vi "cm2nm_center_fids_by_mass.vi"(1 "Array 2":i32[](array[numeric]), 2 "CollectionOfPoints":T1[](array[typedef])) -> (0 "Centered and Scaled":cluster{"X":dbl, "Y":dbl, "Z":dbl}[](array[cluster]))   [LabVIEW 2011]
doc: "Center of mass of the fiducials on the origin and scale by the distance from the origin to the furthest fiducial. Could have alternatively fit to a circle but possibly the fiducials will be not be on a circumference of a circle."
uses:
  cm2nm_coordinate_information_v2.ctl
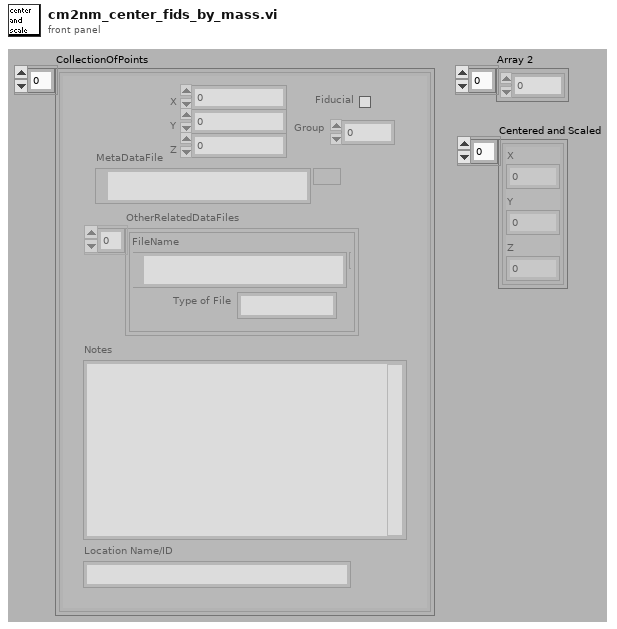
[diagram p1: front panel]
types:
  T1 = typedef "cm2nm_coordinate_information_v2.ctl" = cluster{"MetaDataFile":path, "X":dbl, "Y":dbl, "Z":dbl, "Group":i32, "Rotation":dbl[unit], "Fiducial":bool, "Magnification":dbl, "Working_Distance":dbl, "Notes":string, "Location Name/ID":string, "OtherRelatedDataFiles":cluster{"Type of File":string, "FileName":path}[], "Available":bool}
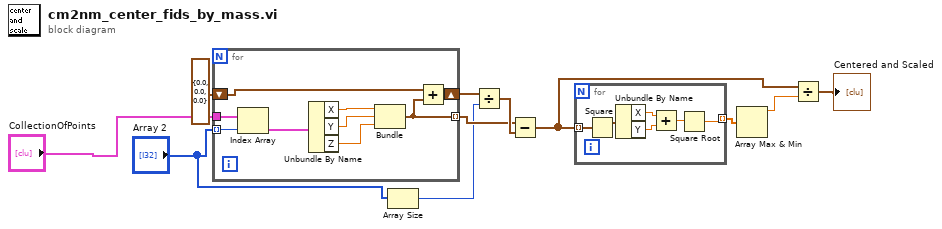
[diagram p0: block diagram]
diagram:
  n1 = for {
    tunnel: "CollectionOfPoints" -> [w20]
    tunnel: "Array 2" -> [w19] mode=indexing
    tunnel: [w14] -> w10 mode=indexing
    shift-right: [w13] -> w7
    shift-left: cluster{"X":dbl, "Y":dbl, "Z":dbl} {"X"=0.0, "Y"=0.0, "Z"=0.0} -> [w12]
    n2 = Index Array(array=w20, index=w19) -> (element=w18:T1)
    n3 = Unbundle By Name(w18) -> ("X"=w17:dbl, "Y"=w16:dbl, "Z"=w15:dbl)
    n4 = Bundle("X"=w17, "Y"=w16, "Z"=w15) -> (w14:cluster{"X":dbl, "Y":dbl, "Z":dbl})  [unwired: 1 out]
    n5 = Add(x=w12, y=w14) -> (x+y=w13:cluster{"X":dbl, "Y":dbl, "Z":dbl})
  }
  n6 = Array Size(array="Array 2") -> (size(s)=w9:i32)
  n7 = Divide(x=w7, y=w9) -> (x/y=w11:cluster{"X":dbl, "Y":dbl, "Z":dbl})
  n8 = Subtract(x=w10, y=w11) -> (x-y=w2:cluster{"X":dbl, "Y":dbl, "Z":dbl}[])
  n9 = for {
    tunnel: w2 -> [w26] mode=indexing
    tunnel: [w21] -> w4 mode=indexing
    n10 = Square(x=w26) -> (x^2=w25:cluster{"X":dbl, "Y":dbl, "Z":dbl})
    n11 = Unbundle By Name(w25) -> ("X"=w24:dbl, "Y"=w23:dbl)
    n12 = Add(x=w24, y=w23) -> (x+y=w22:dbl)
    n13 = Square Root(x=w22) -> (sqrt(x)=w21:dbl)
  }
  n14 = Array Max & Min(array=w4) -> (max value=w3:dbl)  [unwired: 3 out]
  n15 = Divide(x=w2, y=w3) -> (x/y=→"Centered and Scaled":cluster{"X":dbl, "Y":dbl, "Z":dbl}[])
